vi "Advance past whitespace and comments.vi"(4 "Past Colon":bool, 6 "Past Comma":bool, 7 "JSON":string, 9 "Offset":i32, 11 "Parser State in":T1=enum."Leading Whitespace") -> (1 "Offset of first non-whitespace":i32, 3 "Parser State":T1)   [LabVIEW 2019, in "JSONtext.lvlib"]
uses:
  JSONtext.lvlib
  Parsing/Parsing State.ctl
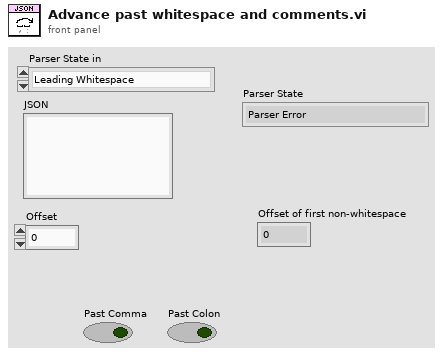
[diagram p1: front panel]
types:
  T1 = typedef "JSONtext.lvlib/Parsing State.ctl" = enum16{"Parser Error", "Object", "Array", "String", "Number/Other", "Leading Whitespace", "Object end", "Array end", "Value end"}
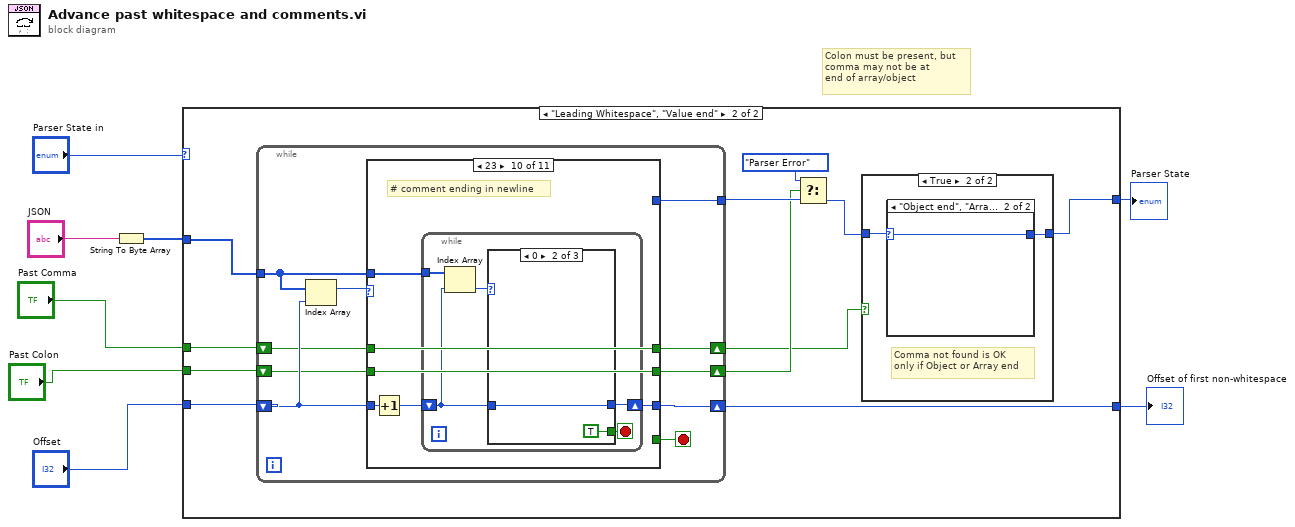
[diagram p0: block diagram]
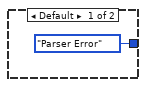
[diagram p4: hidden frame]
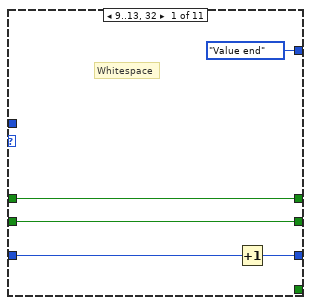
[diagram p5: hidden frame]
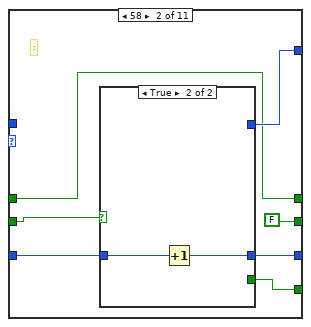
[diagram p6: hidden frame]
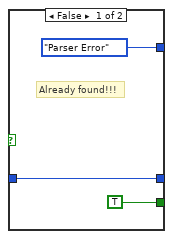
[diagram p7: hidden frame]
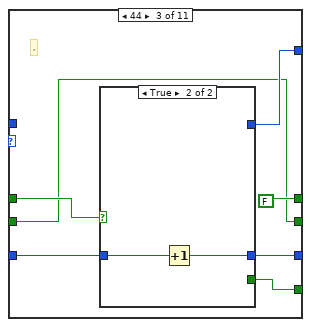
[diagram p8: hidden frame]
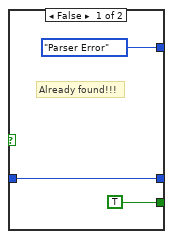
[diagram p9: hidden frame]
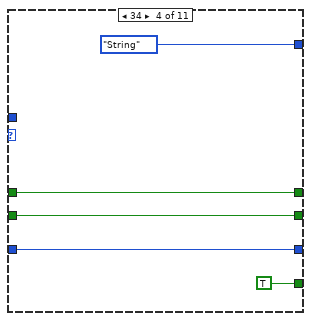
[diagram p10: hidden frame]
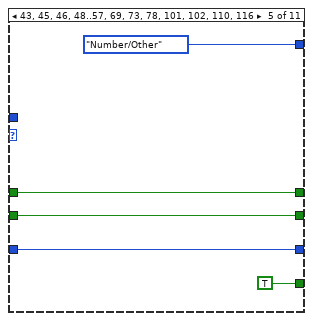
[diagram p11: hidden frame]
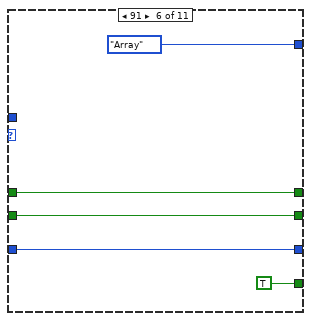
[diagram p12: hidden frame]
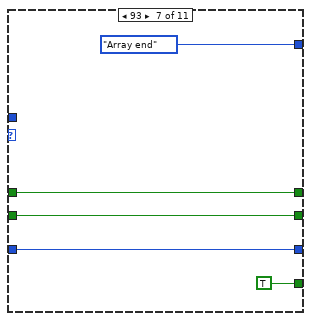
[diagram p13: hidden frame]
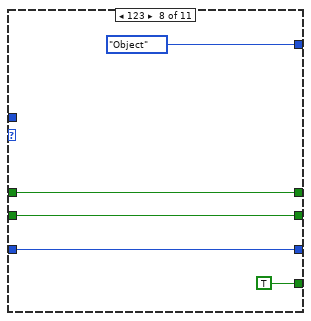
[diagram p14: hidden frame]
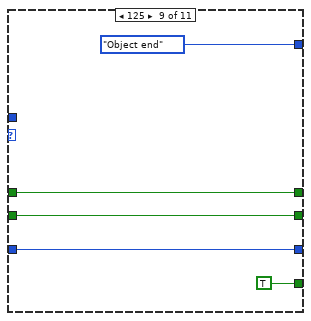
[diagram p15: hidden frame]
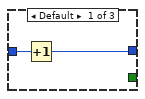
[diagram p16: hidden frame]
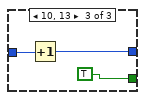
[diagram p17: hidden frame]
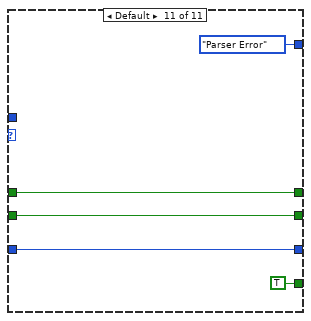
[diagram p18: hidden frame]
diagram:
  # "Colon must be present, but\ncomma may not be at\nend of array/object"
  n1 = String To Byte Array(string="JSON") -> (unsigned byte array=w2:u8[])
  n2 = case shown="\"Leading Whitespace\", \"Value end\"" "Parser State in" {
    selector: "Parser State in" -> [w10 _]
    tunnel: [w10 w21] -> w8
    tunnel: [w9 w20] -> w7
    tunnel: "Offset" -> [w9 w19]
    tunnel: w2 -> [_ w11]
    tunnel: "Past Comma" -> [_ w18]
    tunnel: "Past Colon" -> [_ w17]
    frame "Parser Error", Default {
    }
    frame "Leading Whitespace", "Value end" {
      n3 = while {
        tunnel: w11 -> [w27]
        shift-right: [w32] -> w20
        shift-left: w19 -> [w33]
        tunnel: [w35] -> w16
        shift-right: [w31] -> w13
        shift-left: w18 -> [w30]
        shift-right: [w28] -> w14
        shift-left: w17 -> [w29]
        stop <- w34 stop-if-true
        n4 = Index Array(array=w27, index=w33) -> (element=w36:u8)
        n5 = case shown="23" w36 {
          tunnel: [Parsing_State."Value end" w46 w58 Parsing_State."String" Parsing_State."Number/Other" Parsing_State."Array" Parsing_State."Array end" Parsing_State."Object" Parsing_State."Object end" _ Parsing_State."Parser Error"] -> w35
          tunnel: [_ w45 w57 TRUE TRUE TRUE TRUE TRUE TRUE _ TRUE] -> w34
          tunnel: w33 -> [w41 w48 w60 w68 w73 w78 w83 w88 w93 w101 w118]
          tunnel: [w40 w47 w59 w68 w73 w78 w83 w88 w93 w96 w118] -> w32
          tunnel: [w38 w42 FALSE ("Allow Comma") w67 w72 w77 w82 w87 w92 w100 w115] -> w31
          tunnel: w30 -> [w38 w42 w56 w67 w72 w77 w82 w87 w92 w100 w115]
          tunnel: [w37 FALSE ("Allow Comma") w54 w66 w71 w76 w81 w86 w91 w99 w114] -> w28
          tunnel: w29 -> [w37 w44 w54 w66 w71 w76 w81 w86 w91 w99 w114]
          tunnel: w27 -> [_ _ _ _ _ _ _ _ _ w98 _]
          frame 9..13, 32 {
            # "Whitespace"
            n6 = Increment(x=w41) -> (x+1=w40:i32)
          }
          frame 58 {
            # ":"
            n7 = case shown="True" w44 {
              tunnel: w48 -> [w50 w53]
              tunnel: [w50 w52] -> w47
              tunnel: [Parsing_State."Parser Error" _] -> w46
              tunnel: [TRUE _] -> w45
              frame False {
                # "Already found!!!"
              }
              frame True {
                n8 = Increment(x=w53) -> (x+1=w52:i32)
              }
            }
          }
          frame 44 {
            # ","
            n9 = case shown="True" w56 {
              tunnel: w60 -> [w62 w65]
              tunnel: [w62 w64] -> w59
              tunnel: [Parsing_State."Parser Error" _] -> w58
              tunnel: [TRUE _] -> w57
              frame False {
                # "Already found!!!"
              }
              frame True {
                n10 = Increment(x=w65) -> (x+1=w64:i32)
              }
            }
          }
          frame 34 {
          }
          frame 43, 45, 46, 48..57, 69, 73, 78, 101, 102, 110, 116 {
          }
          frame 91 {
          }
          frame 93 {
          }
          frame 123 {
          }
          frame 125 {
          }
          frame 35 {
            # "# comment ending in newline"
            n11 = Increment(x=w101) -> (x+1=w97:i32)
            n12 = while {
              tunnel: w98 -> [w106]
              shift-right: [w102] -> w96
              shift-left: w97 -> [w104]
              stop <- w103 stop-if-true
              n13 = Index Array(array=w106, index=w104) -> (element=w105:u8)
              n14 = case shown="0" w105 {
                tunnel: w104 -> [w108 w110 w112]
                tunnel: [_ TRUE TRUE] -> w103
                tunnel: [w107 w110 w111] -> w102
                frame Default {
                  n15 = Increment(x=w108) -> (x+1=w107:i32)
                }
                frame 0 {
                }
                frame 10, 13 {
                  n16 = Increment(x=w112) -> (x+1=w111:i32)
                }
              }
            }
          }
          frame Default {
          }
        }
      }
      n17 = Select(t=Parsing_State."Parser Error", s=w14, f=w16) -> (s? t:f=w12:T1)
      n18 = case shown="True" w13 {
        tunnel: w12 -> [w22 w24]
        tunnel: [w22 w23] -> w21
        frame False {
        }
        frame True {
          # "Comma not found is OK\nonly if Object or Array end"
          n19 = case shown="\"Object end\", \"Array end\"" w24 {
            selector: w24 -> [_ w26]
            tunnel: [Parsing_State."Parser Error" w26] -> w23
            frame Default {
            }
            frame "Object end", "Array end" {
            }
          }
        }
      }
    }
  }
  "Parser State" <- w8
  "Offset of first non-whitespace" <- w7
